vi "Write eTestType.vi"(8 "error in (no error)":errorcluster, 10 "eTestType":T1(ring), 11 "PmuAnalysis in":refnum<class "PmuAnalysis.lvclass">) -> (0 "error out":errorcluster, 3 "PmuAnalysis out":refnum<class "PmuAnalysis.lvclass">)   [LabVIEW 2014, in "AnalysisPlugins.lvlib" / "PmuAnalysis.lvclass"]
uses:
  PmuAnalysis.lvclass
  PmuAnalysis.lvclass/PmuAnalysis.ctl
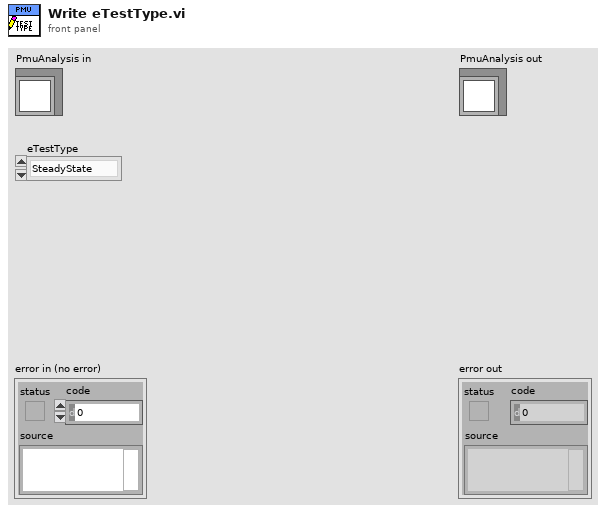
[diagram p1: front panel]
types:
  T1 = enum16{"SteadyState", "Modulation", "Ramp", "Step"}
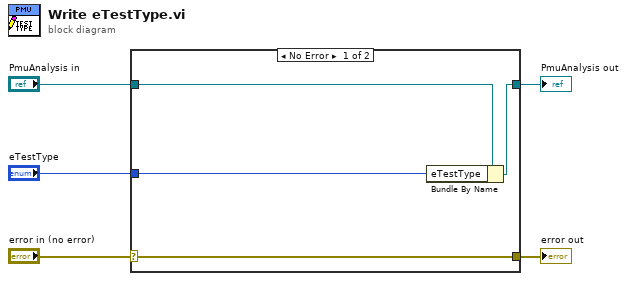
[diagram p0: block diagram]
diagram:
  n1 = case shown="No Error" "error in (no error)" {
    selector: "error in (no error)" -> [w9 w10]
    tunnel: [w9 w10] -> w4
    tunnel: [w7 w11] -> w2
    tunnel: "PmuAnalysis in" -> [w8 w11]
    tunnel: "eTestType" -> [w6 _]
    frame No Error {
      n2 = Bundle By Name(cluster=w8, "eTestType"=w6) -> (w7:refnum<class "PmuAnalysis.lvclass">)
    }
    frame Error {
    }
  }
  "error out" <- w4
  "PmuAnalysis out" <- w2
